vi "Initialize Buffer Converter.vi"(8 "error in (no error)":errorcluster, 9 "Transfer Groups":refnum<class "Transfer Group.lvclass">[](array[class]), 10 "component classes":refnum<class>[](array[class]), 11 "Plugin in":refnum<class "Plugin.lvclass">) -> (0 "error out":errorcluster, 2 "Buffer Converter":refnum<class "Buffer Converter.lvclass">, 3 "Plugin out":refnum<class "Plugin.lvclass">)   [LabVIEW 2017, in "DSF Core.lvlib" / "Plugin.lvclass"]
uses:
  Plugin.lvclass
  Buffer Converter/Buffer Converter.lvclass
  Transfer Group/Transfer Group.lvclass
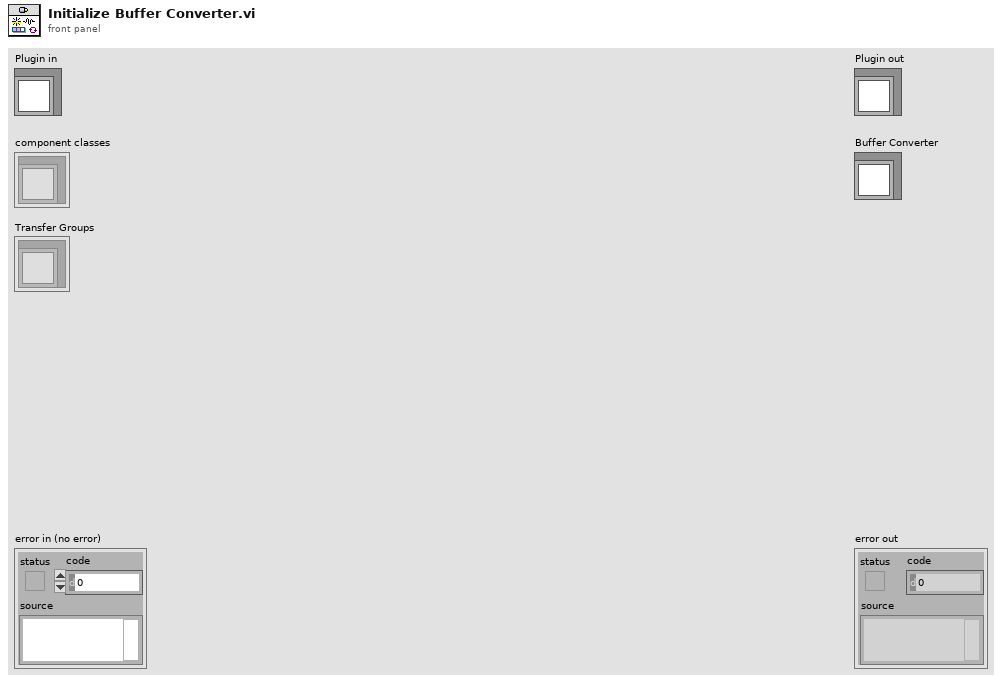
[diagram p1: front panel]
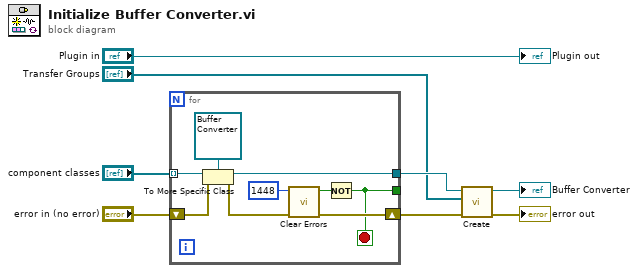
[diagram p0: block diagram]
diagram:
  n1 = for {
    tunnel: "component classes" -> [w16] mode=indexing
    shift-right: [w13] -> w3
    shift-left: "error in (no error)" -> [w12]
    tunnel: [w10] -> _
    tunnel: [w9] -> w5
    stop <- w10 stop-if-true
    n2 = To More Specific Class(target class=refnum<class "Buffer Converter.lvclass"> refnum ("DSF.Engine.lvlib:Transceiver"), reference=w16, error in=w12) -> (specific class reference=w9:refnum<class "Buffer Converter.lvclass">, error out=w14:errorcluster)
    n3 = call <vilib>:"Clear Errors.vi"("error in (no error)"=w14, "specific error code to clear (0: all)"=1448) -> ("error out"=w13:errorcluster, "specific error cleared?"=w11:bool)  [unwired: 4 in]
    n4 = Not(x=w11) -> (.not. x?=w10:bool)
  }
  n5 = call "Create.vi"("error in (no error)"=w3, "Transfer Groups"="Transfer Groups", "Buffer Converter type"=w5) -> ("error out"=→"error out":errorcluster, "Buffer Converter out"=→"Buffer Converter":refnum<class "Buffer Converter.lvclass">)  [unwired: 7 in]
  "Plugin out" <- "Plugin in"
